vi "Occurrence Speed Counter.vi"(8 "period(0.1s)":dbl=0.1, 11 "Occured?(T)":bool=TRUE) -> (0 "New?":bool, 2 "Last Check Time":timestamp, 3 "Speed(#/s)":dbl)   [LabVIEW 2017, in "Communicable State Machine.lvlib"]
uses:
  Communicable State Machine.lvlib
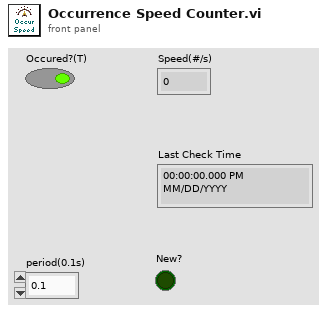
[diagram p1: front panel]
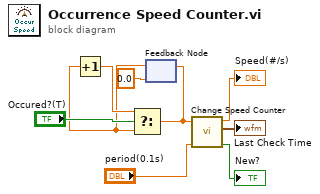
[diagram p0: block diagram]
diagram:
  n1 = feedback #1(0.0) -> (w4:dbl)
  n2 = Increment(x=w4) -> (x+1=w8:dbl)
  n3 = Select(t=w8, s="Occured?(T)", f=w4) -> (s? t:f=w3:dbl)
  n4 = feedback-in #1(w3) -> ()
  n5 = call "Change Speed Counter.vi"("period(0.1s)"="period(0.1s)", "Numeric"=w3) -> ("New?"=→"New?":bool, "Last Check Time"=→"Last Check Time":timestamp, "Speed(#/s)"=→"Speed(#/s)":dbl)  [unwired: 7 in]
